vi "Demo test 1.vi"(0 "vi path":path=path "D:/SLL Drona/Prototype/Issue 35 - Subpanel load Error/Demo VI.vi", 11 "error in":errorcluster) -> (3 "VI Ref same?":bool, 4 "VI Name":string, 15 "error out":errorcluster)   [LabVIEW 2016]
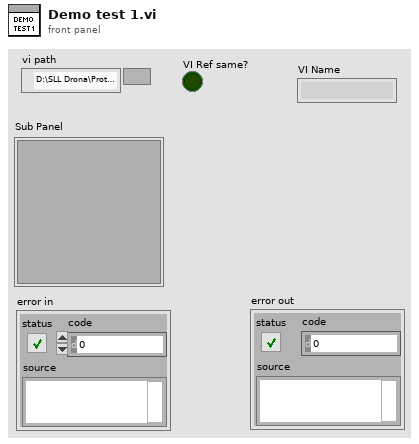
[diagram p1: front panel]
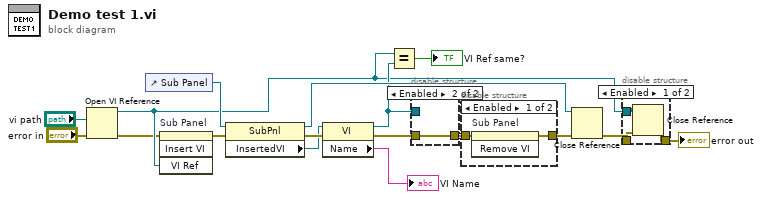
[diagram p0: block diagram]
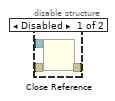
[diagram p3: hidden frame]
diagram:
  n1 = Open VI Reference(vi path="vi path", error in (no error)="error in") -> (vi reference=w5:refnum<vi>, error out=w2:errorcluster)  [unwired: 4 in]
  n2 = control-ref of="Sub Panel"() -> (w16:refnum<vi>)
  n3 = invoke on="Sub Panel" class="SubPnl" method="Insert VI"(error in=w2, "VI Ref"=w5) -> (error out=w7:errorcluster)  [unwired: 2 in, 3 out]
  n4 = property class="SubPnl"(reference=w16, error in=w7) -> (reference out=w9:refnum<vi>, error out=w14:errorcluster, "InsertedVI"=w8:refnum<vi>)
  n5 = property class="VI"(reference=w8, error in=w14) -> (reference out=w6:refnum<vi>, error out=w13:errorcluster, "Name"=→"VI Name":string)
  n6 = Equal?(x=w5, y=w6) -> (x = y?=→"VI Ref same?":bool)
  n7 = disable-structure shown="Enabled" {
    disable-tunnel: w6 -> [w20 _]
    disable-tunnel: w13 -> [w19 w21]
    disable-tunnel: [w18 w21] -> w3
    frame Disabled {
      n8 = Close Reference(reference=w20, error in (no error)=w19) -> (error out=w18:errorcluster)
    }
    frame Enabled {
    }
  }
  n9 = disable-structure shown="Enabled" {
    disable-tunnel: [w23 w24] -> w11
    disable-tunnel: w3 -> [w22 w24]
    frame Enabled {
      n10 = invoke on="Sub Panel" class="SubPnl" method="Remove VI"(error in=w22) -> (error out=w23:errorcluster)  [unwired: 2 in, 2 out]
    }
    frame Disabled {
    }
  }
  n11 = Close Reference(reference=w9, error in (no error)=w11) -> (error out=w12:errorcluster)
  n12 = disable-structure shown="Enabled" {
    disable-tunnel: w12 -> [w27 w28]
    disable-tunnel: [w26 w28] -> w10
    disable-tunnel: w5 -> [w25 _]
    frame Enabled {
      n13 = Close Reference(reference=w25, error in (no error)=w27) -> (error out=w26:errorcluster)
    }
    frame Disabled {
    }
  }
  "error out" <- w10
